vi "Force Recorder.vi"() -> ()   [LabVIEW 2017]
uses:
  <vilib>/Platform/TimedLoop/XDataNode/timing_clust.ctl
  <vilib>/Platform/TimedLoop/XDataNode/nitl_modes.ctl
  <vilib>/Platform/TimedLoop/XDataNode/wakeup.ctl
  <vilib>/Utility/sysdir.llb/System Directory Type.ctl
  <vilib>/DAQmx/read.llb/DAQmx Read (Analog 1D DBL NChan 1Samp).vi
  <vilib>/Instr/_visa.llb/VISA Configure Serial Port (Instr).vi
  <vilib>/Utility/file.llb/Write Delimited Spreadsheet (string).vi
  <vilib>/Utility/file.llb/Write Delimited Spreadsheet (DBL).vi
  <vilib>/DAQmx/create/channels.llb/DAQmx Create Channel (AI-Voltage-Basic).vi
  <vilib>/DAQmx/configure/timing.llb/DAQmx Timing (Sample Clock).vi
  <vilib>/DAQmx/miscellaneous.llb/DAQmx Fill In Error Info.vi
  <vilib>/platform/TimedLoop/XDataNode/XDataNode.xnode
  <vilib>/Platform/TimedLoop/XDataNode/XDNodeRunTimeDep.lvlib
panel:
  out "FW Up":i32
  out "RW Down":i32
  out "RW Up":i32
  out "FW Down":i32
  out "Loop":i32
  out "Save in Time":dbl[][](array[numeric])
  out "SaveReady":bool
  out "RW Force Up":T1
  out "FW Force Up":T1
  out "RW Force Down":T1
  out "FW Force Down":T1
  in  "Read":bool
  in  "Save Type":enum32{"Save in time", "Save by step force"}(radio) caption="Save By Step Force"
  out "Volt Meter 2":dbl(graph)=0.034576825000000005
  in  "SAVE":bool
  out "Save Path":path
  out "Volt Meter 1":dbl(graph)=0.0048819160000000035
  in  "Test Name":string(combo)="DL"
  in  "Lane Number":string(combo)="Lane 1"
  out "Force Meter":dbl(graph)=0.06621116599999999
  out "error out":errorcluster
  in  "stop":bool
  out "Serial OK":bool
  out "Step Force":u8[](array[numeric])
  in  "Serial Port":refnum<visa-resource-name>="COM3"
  in  "Baud Rate":string(combo)="19200"
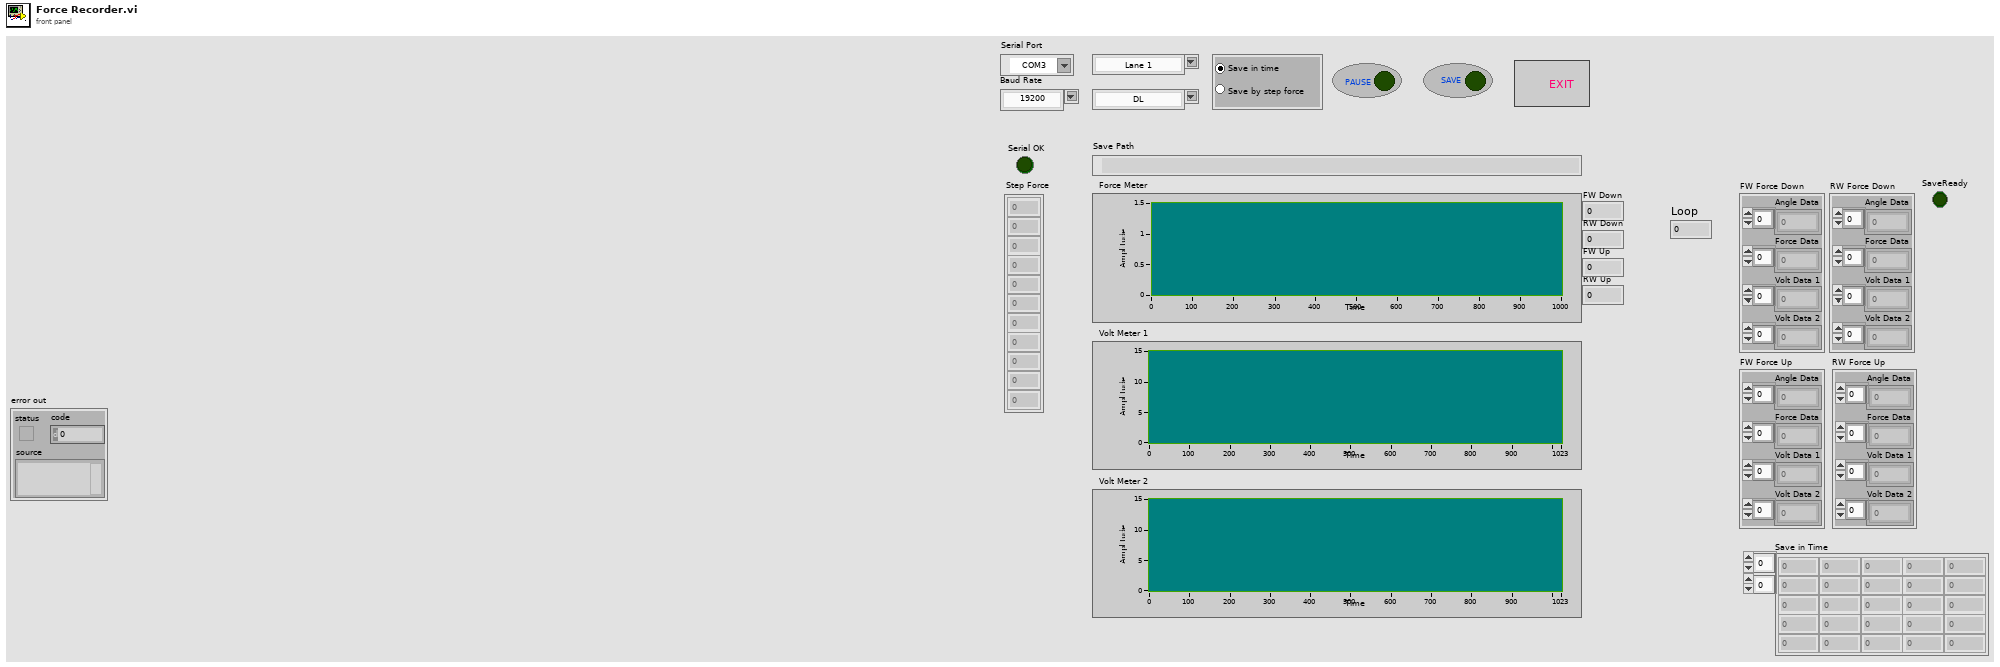
[diagram p1: front panel]
types:
  T1 = cluster{"Angle Data":dbl[], "Force Data":dbl[], "Volt Data 1":dbl[], "Volt Data 2":dbl[]}
  T2 = cluster{"Angle":dbl[], "Force":dbl[], "Volt 1":dbl[], "Volt 2":dbl[]}
  T3 = typedef "XDNodeRunTimeDep.lvlib/timing_clust.ctl" = cluster{"Expected End [f-1]":u64, "Actual End [f-1]":u64, "Finished Late? [f-1]":bool, "Expected End [i-1]":u64, "Actual End [i-1]":u64, "Finished Late? [i-1]":bool, "Expected Start [i]":u64, "Actual Start [i]":u64, "Expected Start [f]":u64, "Actual Start [f]":u64, "Source Name":string, "Structure Name":string, "Period":i64, "Deadline":i64, "Offset":i64, "Start":i64, "Priority":i32, "Timeout":i32, "Mode":T4, "Wakeup Reason":T5, "Error":errorcluster, "Source Type":string, "Secondary Source Type":string, "Global End Time":u64, "Global Start Time":u64, "Frame Duration":u64, "Iteration Duration":u64, "Assigned CPU":i32, "I/O Scan Engine Mode":u32}
  T4 = typedef "XDNodeRunTimeDep.lvlib/nitl_modes.ctl" = enum32{"No Change", "Process missed periods, maintain original phase", "Discard missed periods, maintain original phase", "Process missed periods, ignore original phase", "Discard missed periods, ignore original phase"}
  T5 = typedef "XDNodeRunTimeDep.lvlib/wakeup.ctl" = enum32{"Normal", "Aborted", "Asynchronous wakeup", "Timing source error", "Timed loop error", "Timeout"}
  T6 = enum8{"Enabled", "Disabled", "Disabled and Grayed Out"}
  T7 = typedef "System Directory Type.ctl" = i32
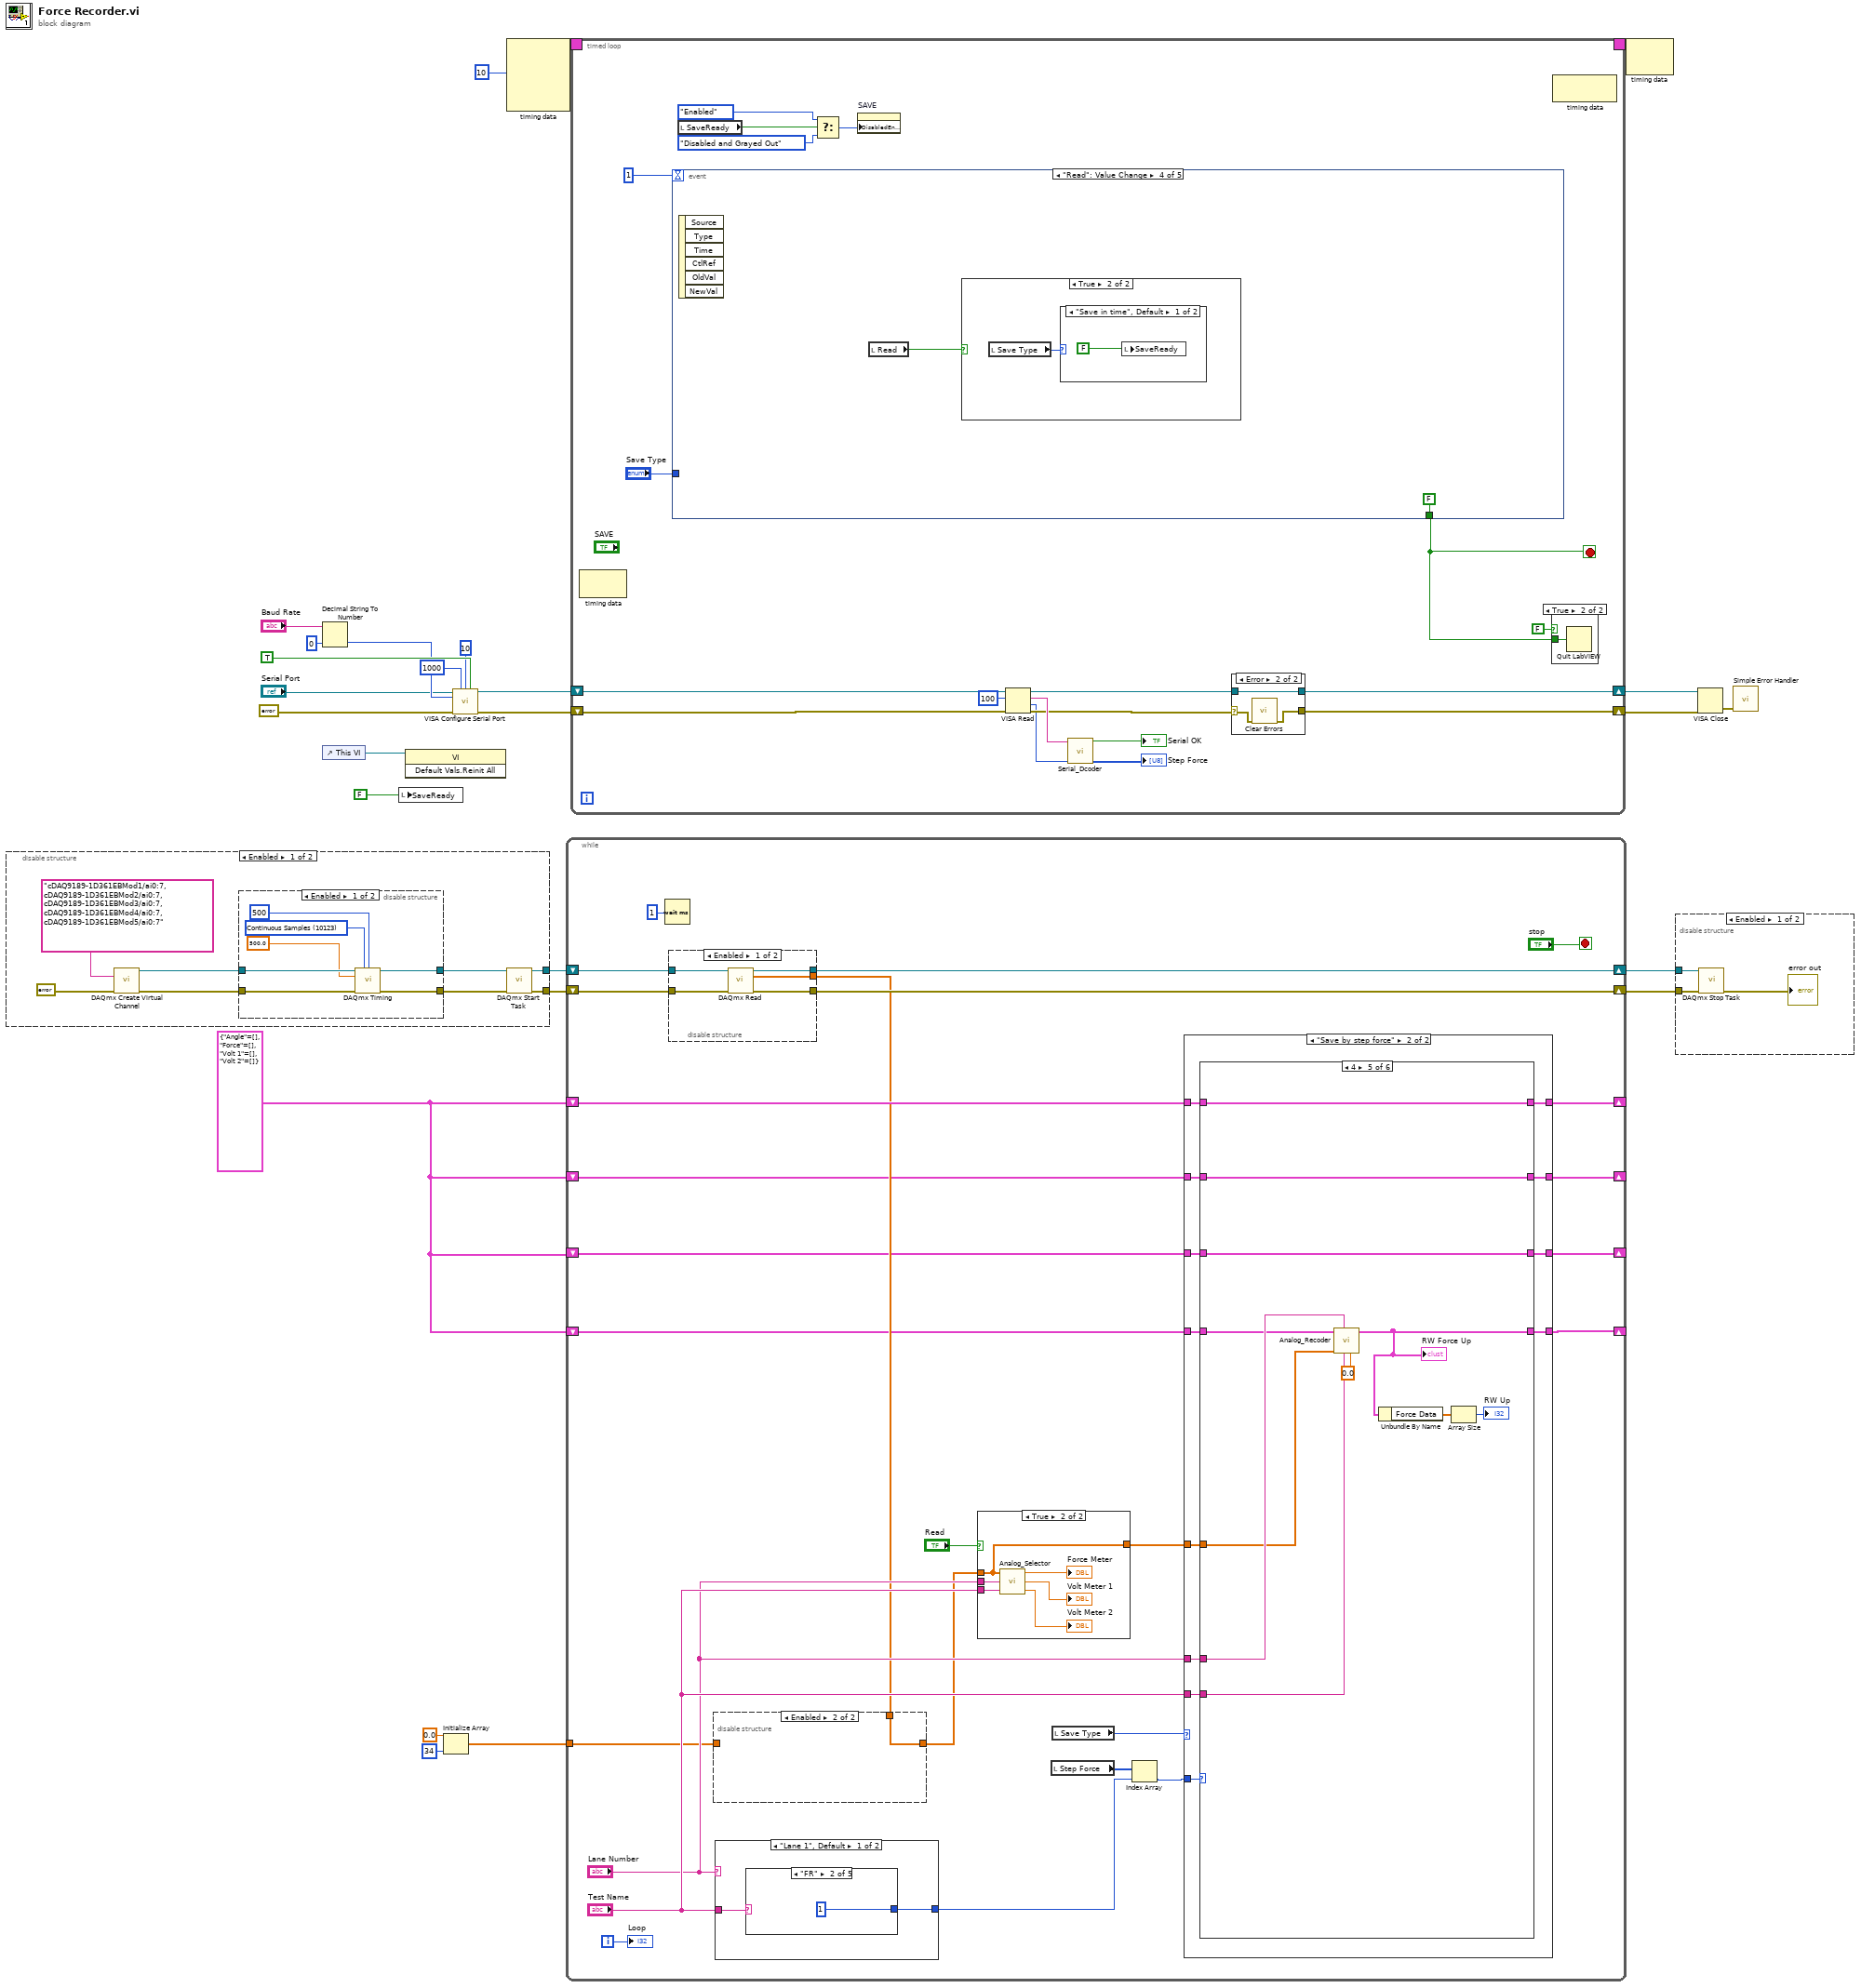
[diagram p0: block diagram]
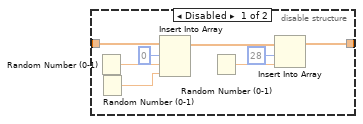
[diagram p2: hidden frame]
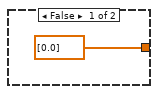
[diagram p3: hidden frame]
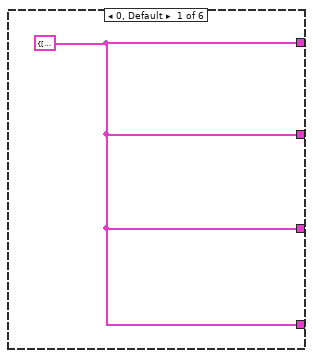
[diagram p5: hidden frame]
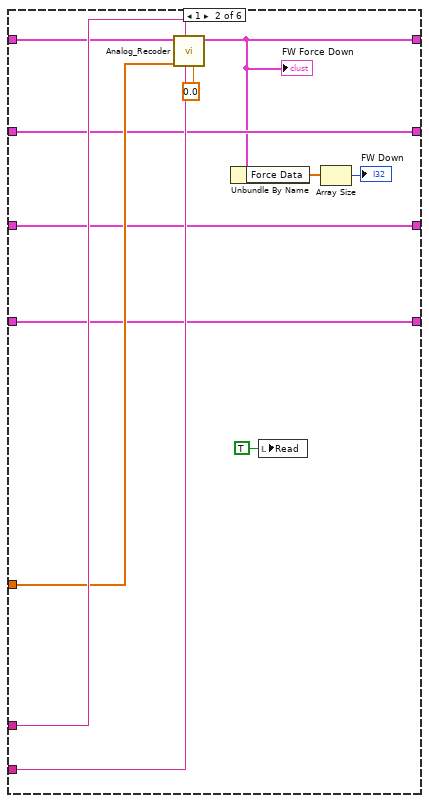
[diagram p6: hidden frame]
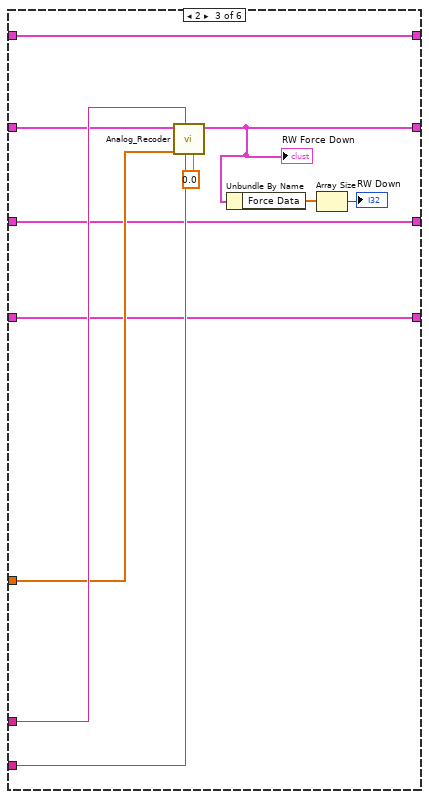
[diagram p7: hidden frame]
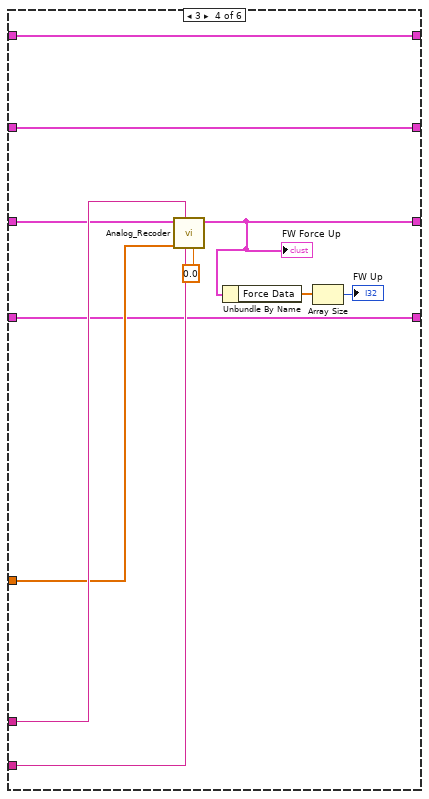
[diagram p8: hidden frame]
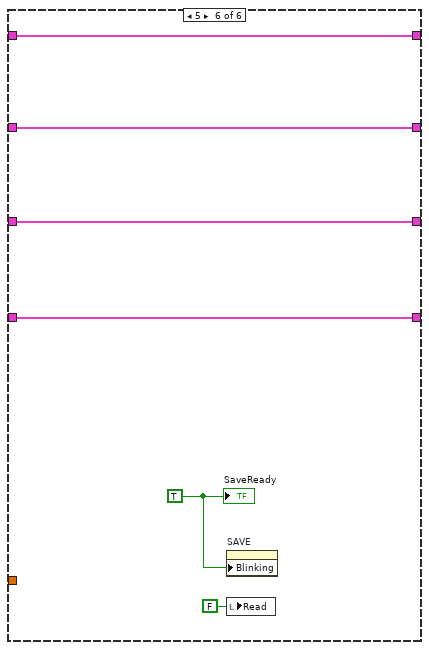
[diagram p9: hidden frame]
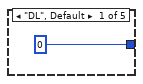
[diagram p11: hidden frame]
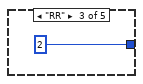
[diagram p12: hidden frame]
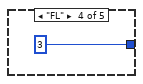
[diagram p13: hidden frame]
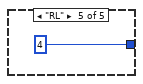
[diagram p14: hidden frame]
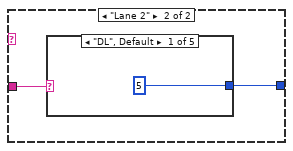
[diagram p15: hidden frame]
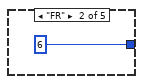
[diagram p16: hidden frame]
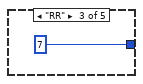
[diagram p17: hidden frame]
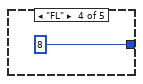
[diagram p18: hidden frame]
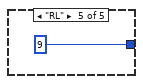
[diagram p19: hidden frame]
diagram:
  w2 = T2 {"Angle"=[], "Force"=[], "Volt 1"=[], "Volt 2"=[]}
  n1 = disable-structure shown="Enabled" {
    disable-tunnel: [w34 _] -> w9
    disable-tunnel: [w33 _] -> w8
    frame Enabled {
      n2 = call-poly <vilib>:"DAQmx Create Virtual Channel.vi"("physical channels"=tag "cDAQ9189-1D361EBMod1/ai0:7, cDAQ9189-1D361EBMod2/ai0:7, cDAQ9189-1D361EBMod3/ai0:7, cDAQ9189-1D361EBMod4/ai0:7, cDAQ9189-1D361EBMod5/ai0:7", "error in"=errorcluster {"status"=FALSE, "code"=0, "source"=""} ("error constant")) -> ("task out"=w30:refnum<k21>, "error out"=w29:errorcluster)  [unwired: 12 in]
      n3 = disable-structure shown="Enabled" {
        disable-tunnel: w30 -> [w41 w43]
        disable-tunnel: w29 -> [w40 w42]
        disable-tunnel: [w39 w43] -> w28
        disable-tunnel: [w38 w42] -> w27
        frame Enabled {
          w36 = 10123 items=["Finite Samples"=10178, "Continuous Samples"=10123, "Hardware Timed Single Point"=12522] ("sample mode")
          n4 = call-poly <vilib>:"DAQmx Timing.vi"("task/channels in"=w41, "sample mode"=w36, "samples per channel"=500, "rate"=500.0, "error in"=w40) -> ("task out"=w39:refnum<k21>, "error out"=w38:errorcluster)  [unwired: 9 in]
        }
        frame Disabled {
        }
      }
      n5 = call <vilib>:"DAQmx Start Task.vi"("task/channels in"=w28, "error in"=w27) -> ("task out"=w34:refnum<k21>, "error out"=w33:errorcluster)  [unwired: 12 in]
    }
    frame Disabled {
    }
  }
  n6 = Decimal String To Number(string="Baud Rate", default (0L)=u32 0 ("default (0 I32)")) -> (number=w18:u32)  [unwired: 1 in, 1 out]
  n7 = control-ref of="This VI"() -> (w10:refnum<vi>)
  n8 = local write "SaveReady"(FALSE ("SaveReady")) -> ()
  n9 = invoke class="VI" method="Default Vals.Reinit All"(reference=w10) -> ()  [unwired: 2 in, 3 out]
  n10 = Initialize Array(0.0 ("element"), 34 ("dimension size")) -> (w3:dbl[])
  n11 = call-poly "VISA Configure Serial Port"("VISA resource name"="Serial Port", "timeout (10sec)"=u32 1000, "termination char\n(0xA = '\\n' = LF)"=u8 10 ("termination char\n(0xA = '\\n' = LF)"), "Enable Termination\nChar (T)"=TRUE ("End Read on Termination Character?"), "baud rate (9600)"=w18, "error in (no error)"=errorcluster {"status"=FALSE, "code"=0, "source"=""}) -> ("VISA resource name out"=w16:refnum<visa-resource-name>, "error out"=w15:errorcluster)  [unwired: 4 in, 4 out]
  n12 = node-c288(i64 10 ("Period")) -> (w26:T3)  [unwired: 3 in]
  n13 = while {
    shift-right: [w63] -> w7
    shift-left: w9 -> [w65]
    shift-right: [w62] -> w6
    shift-left: w8 -> [w64]
    shift-right: [w68] -> _
    shift-left: w2 -> [w69]
    tunnel: w3 -> [w58]
    shift-right: [w53] -> _
    shift-left: w2 -> [w52]
    shift-right: [w50] -> _
    shift-left: w2 -> [w51]
    shift-right: [w49] -> _
    shift-left: w2 -> [w48]
    i -> [w47]
    stop <- "stop" stop-if-true
    n14 = Wait (ms)(milliseconds to wait=u32 1) -> ()  [unwired: 1 out]
    n15 = disable-structure shown="Enabled" {
      disable-tunnel: w65 -> [w158 _]
      disable-tunnel: w64 -> [w157 _]
      disable-tunnel: [w156 _] -> w63
      disable-tunnel: [w155 _] -> w62
      disable-tunnel: [w154 _] -> w55
      frame Enabled {
        n16 = call-poly <vilib>:"DAQmx Read.vi"("task/channels in"=w158, "error in"=w157) -> ("task out"=w156:refnum<k21>, "data"=w154:dbl[], "error out"=w155:errorcluster)  [unwired: 11 in]
      }
      frame Disabled {
      }
    }
    n17 = disable-structure shown="Enabled" {
      disable-tunnel: w58 -> [w73 _]
      disable-tunnel: [w70 w78] -> w56
      disable-tunnel: w55 -> [_ w78]
      frame Disabled {
        n18 = Random Number (0-1)() -> (number: 0 to 1=w75:dbl)
        n19 = Random Number (0-1)() -> (number: 0 to 1=w71:dbl)
        n20 = Insert Into Array(array=w73, index=0, new element #1=w75, new element #2=w71) -> (w72:dbl[])
        n21 = Random Number (0-1)() -> (number: 0 to 1=w76:dbl)
        n22 = Insert Into Array(array=w72, index=28, new element=w76) -> (w70:dbl[])
      }
      frame Enabled {
      }
    }
    n23 = case shown="\"Lane 1\", Default" "Lane Number" {
      tunnel: "Test Name" -> [w160 w167]
      tunnel: [w159 w166] -> w67
      frame "Lane 1", Default {
        n24 = case shown="\"FR\"" w160 {
          tunnel: [0 ("index") 1 ("index") 2 ("index") 3 ("index") 4 ("index")] -> w159
          frame "DL", Default {
          }
          frame "FR" {
          }
          frame "RR" {
          }
          frame "FL" {
          }
          frame "RL" {
          }
        }
      }
      frame "Lane 2" {
        n25 = case shown="\"DL\", Default" w167 {
          tunnel: [5 ("index") 6 ("index") 7 ("index") 8 ("index") 9 ("index")] -> w166
          frame "DL", Default {
          }
          frame "FR" {
          }
          frame "RR" {
          }
          frame "FL" {
          }
          frame "RL" {
          }
        }
      }
    }
    n26 = case shown="True" "Read" {
      tunnel: "Test Name" -> [_ w82]
      tunnel: "Lane Number" -> [_ w81]
      tunnel: w56 -> [_ w80]
      tunnel: [dbl[] [0.0] w80] -> w54
      frame False {
      }
      frame True {
        n27 = call "Analog_Selector.vi"("Test Name"=w82, "Lane Number"=w81, "Analog Data In"=w80) -> ("Volt 2"=→"Volt Meter 2":dbl, "Volt 1"=→"Volt Meter 1":dbl, "Force"=→"Force Meter":dbl)
      }
    }
    n28 = local read "Step Force"() -> (w66:u8[])
    n29 = local read "Save Type"() -> (w59:enum32{"Save in time", "Save by step force"})
    n30 = Index Array(array=w66, index=w67) -> (element=w44:u8)
    n31 = case shown="\"Save by step force\"" w59 {
      tunnel: w69 -> [w89 w101]
      tunnel: [w89 w100] -> w68
      tunnel: w54 -> [_ w99]
      tunnel: w44 -> [_ w98]
      tunnel: "Test Name" -> [_ w97]
      tunnel: "Lane Number" -> [_ w96]
      tunnel: [w88 w95] -> w53
      tunnel: w52 -> [w88 w94]
      tunnel: w51 -> [w87 w93]
      tunnel: [w87 w92] -> w50
      tunnel: [w86 w91] -> w49
      tunnel: w48 -> [w86 w90]
      frame "Save in time", Default {
      }
      frame "Save by step force" {
        n32 = case shown="4" w98 {
          tunnel: w101 -> [_ w111 w118 w131 w143 w153]
          tunnel: [w102 w105 w118 w131 w143 w153] -> w100
          tunnel: w99 -> [_ w112 w123 w134 w145 _]
          tunnel: w97 -> [_ w113 w124 w135 w146 _]
          tunnel: w96 -> [_ w114 w125 w136 w147 _]
          tunnel: [w102 w109 w115 w129 w142 w152] -> w95
          tunnel: w94 -> [_ w109 w119 w129 w142 w152]
          tunnel: [w102 w108 w121 w126 w141 w151] -> w92
          tunnel: w93 -> [_ w108 w121 w130 w141 w151]
          tunnel: [w102 w107 w120 w132 w137 w150] -> w91
          tunnel: w90 -> [_ w107 w120 w132 w140 w150]
          frame 0, Default {
            w102 = T2 {"Angle"=[], "Force"=[], "Volt 1"=[], "Volt 2"=[]}
          }
          frame 1 {
            n33 = call "Analog_Recoder.vi"("External Angle In"=0.0, "Test Name"=w113, "Lane Number"=w114, "Analog Data In"=w112, "Analog Array In"=w111) -> ("Analog Array Out"=w105:T1)  [unwired: 6 in]
            "FW Force Down" <- w105
            n34 = Unbundle By Name(w105) -> ("Force Data"=w104:dbl[])
            n35 = local write "Read"(TRUE ("Read")) -> ()
            n36 = Array Size(array=w104) -> (size(s)=→"FW Down":i32)
          }
          frame 2 {
            n37 = call "Analog_Recoder.vi"("External Angle In"=0.0, "Test Name"=w124, "Lane Number"=w125, "Analog Data In"=w123, "Analog Array In"=w119) -> ("Analog Array Out"=w115:T1)  [unwired: 6 in]
            "RW Force Down" <- w115
            n38 = Unbundle By Name(w115) -> ("Force Data"=w117:dbl[])
            n39 = Array Size(array=w117) -> (size(s)=→"RW Down":i32)
          }
          frame 3 {
            n40 = call "Analog_Recoder.vi"("External Angle In"=0.0, "Test Name"=w135, "Lane Number"=w136, "Analog Data In"=w134, "Analog Array In"=w130) -> ("Analog Array Out"=w126:T1)  [unwired: 6 in]
            "FW Force Up" <- w126
            n41 = Unbundle By Name(w126) -> ("Force Data"=w128:dbl[])
            n42 = Array Size(array=w128) -> (size(s)=→"FW Up":i32)
          }
          frame 4 {
            n43 = call "Analog_Recoder.vi"("External Angle In"=0.0, "Test Name"=w146, "Lane Number"=w147, "Analog Data In"=w145, "Analog Array In"=w140) -> ("Analog Array Out"=w137:T1)  [unwired: 6 in]
            "RW Force Up" <- w137
            n44 = Unbundle By Name(w137) -> ("Force Data"=w139:dbl[])
            n45 = Array Size(array=w139) -> (size(s)=→"RW Up":i32)
          }
          frame 5 {
            w149 = TRUE ("SaveReady")
            n46 = property on="SAVE" class="Bool (strict)"("Blinking"=w149) -> ()  [unwired: 2 in, 2 out]
            n47 = local write "Read"(FALSE ("Read")) -> ()
            "SaveReady" <- w149
          }
        }
      }
    }
    "Loop" <- w47
  }
  n48 = timed-loop {
    timing: w26 -> [_]
    timing-out: [_] -> w25
    shift-right: [w191] -> w14
    shift-left: w16 -> [w184]
    shift-right: [w190] -> w13
    shift-left: w15 -> [w185]
    stop <- w173 stop-if-true
    n49 = node-c288() -> ()  [unwired: 1 in, 1 out]
    n50 = event shown="[3] \"Read\": Value Change" {
      selector: _ -> [_ _ _ _ _]
      dyn-events: _ -> [_ _ _ _ _]
      timeout: 1 -> [_ _ _ _ _]
      tunnel: [FALSE TRUE FALSE FALSE FALSE] -> w173
      tunnel: "Save Type" -> [_ _ w217 _ _]
      event Timeout {
        n51 = event-data() -> ()  [unwired: 1 in, 3 out]
      }
      event "stop": Value Change {
        n52 = event-data() -> ()  [unwired: 1 in, 3 out]
      }
      event "SAVE": Value Change {
        w197 = "_" ("string")
        w216 = T7 1 items=["User Home"=0, "User Desktop"=1, "User Documents"=2, "User Application Data"=3, "User Preferences"=4, "User Temporary"=5, "Public Documents"=6, "Public Application Data"=7, "Public Preferences"=8, "Public Cache"=13, "System Core Libraries"=9, "System Installed Libraries"=10, "Application Files"=11, "Boot Volume Root"=12] ("system directory type")
        n53 = event-data() -> ()  [unwired: 1 in, 6 out]
        n54 = local read "Lane Number"() -> (w205:string)
        n55 = local read "Test Name"() -> (w204:string)
        n56 = local write "SaveReady"(FALSE ("SaveReady")) -> ()
        n57 = Get Date/Time String(date format (0)=enum16{"short", "long", "abbreviated"}."short", want seconds? (F)=TRUE) -> (date string=w210:string, time string=w199:string)  [unwired: 1 in]
        n58 = Search and Replace String(replace all?=TRUE ("replace all? (F)"), input string=w210, search string="/", replace string="-" ("replace string (\"\")")) -> (result string=w206:string)  [unwired: 4 in, 3 out]
        n59 = Search and Replace String(replace all?=TRUE ("replace all? (F)"), input string=w199, search string=":", replace string="") -> (result string=w198:string)  [unwired: 4 in, 3 out]
        n60 = call <vilib>:"Get System Directory.vi"("system directory type"=w216) -> ("system directory"=w215:path)  [unwired: 10 in]
        n61 = Path To String(path=w215) -> (string=w214:string)
        n62 = Concatenate Strings(w214, "\\" ("string"), "ForceLog_" ("string"), w206, w197, w198, w197, w205, w197, w204) -> (w194:string)
        n63 = property on="SAVE" class="Bool (strict)"("Blinking"=FALSE) -> ()  [unwired: 2 in, 2 out]
        n64 = case shown="\"Save by step force\"" w217 {
          tunnel: w194 -> [w219 w243]
          frame "Save in time", Default {
            n65 = stacked-sequence {
              tunnel: w219 -> [w220 w232]
              frame #0 {
                n66 = Concatenate Strings(w220, ".csv" ("string")) -> (w222:string)
                n67 = String To Path(string=w222) -> (path=w221:path)
                n68 = call-poly <vilib>:"Write Delimited Spreadsheet.vi"("file path (dialog if empty)"=w221, "2D data"=string[][] [["Angle", "Force", "Volt 1", "Volt 2"]], "append to file? (new file:F)"=TRUE, "transpose? (no:F)"=FALSE, "delimiter (\\t)"="," ("delimiter (\\t)")) -> ()  [unwired: 9 in, 2 out]
              }
              frame #1 {
                n69 = property on="Force Meter" class="WFChart (strict)"() -> ("History Data"=w236:dbl[])  [unwired: 2 in, 2 out]
                n70 = property on="Volt Meter 1" class="WFChart (strict)"() -> ("History Data"=w235:dbl[])  [unwired: 2 in, 2 out]
                n71 = property on="Volt Meter 2" class="WFChart (strict)"() -> ("History Data"=w234:dbl[])  [unwired: 2 in, 2 out]
                n72 = Concatenate Strings(w232, ".csv" ("string")) -> (w230:string)
                n73 = String To Path(string=w230) -> (path=w229:path)
                n74 = Build Array(dbl[] [0.0] ("element"), w236, w235, w234) -> (w241:dbl[][])
                "Save in Time" <- w241
                n75 = Transpose 2D Array(2D array=w241) -> (transposed array=w242:dbl[][])
                n76 = call-poly <vilib>:"Write Delimited Spreadsheet.vi"("file path (dialog if empty)"=w229, "format (%.3f)"="%.6f", "2D data"=w242, "append to file? (new file:F)"=TRUE, "transpose? (no:F)"=FALSE, "delimiter (\\t)"="," ("delimiter (\\t)")) -> ("new file path (Not A Path if cancelled)"=→"Save Path":path)  [unwired: 8 in, 1 out]
              }
            }
          }
          frame "Save by step force" {
            n77 = stacked-sequence {
              tunnel: w243 -> [w244 w252 w260 w268 w284 w298 w312 w326]
              frame #0 {
                n78 = Concatenate Strings(w244, "_FW_Down.csv" ("string")) -> (w247:string)
                n79 = String To Path(string=w247) -> (path=w245:path)
                n80 = call-poly <vilib>:"Write Delimited Spreadsheet.vi"("file path (dialog if empty)"=w245, "2D data"=string[][] [["Angle", "Force", "Volt 1", "Volt 2"]], "append to file? (new file:F)"=FALSE, "transpose? (no:F)"=FALSE, "delimiter (\\t)"="," ("delimiter (\\t)")) -> ()  [unwired: 9 in, 2 out]
              }
              frame #1 {
                n81 = Concatenate Strings(w252, "_RW_Down.csv" ("string")) -> (w255:string)
                n82 = String To Path(string=w255) -> (path=w253:path)
                n83 = call-poly <vilib>:"Write Delimited Spreadsheet.vi"("file path (dialog if empty)"=w253, "2D data"=string[][] [["Angle", "Force", "Volt 1", "Volt 2"]], "append to file? (new file:F)"=FALSE, "transpose? (no:F)"=FALSE, "delimiter (\\t)"="," ("delimiter (\\t)")) -> ()  [unwired: 9 in, 2 out]
              }
              frame #2 {
                n84 = Concatenate Strings(w260, "_FW_Up.csv" ("string")) -> (w263:string)
                n85 = String To Path(string=w263) -> (path=w261:path)
                n86 = call-poly <vilib>:"Write Delimited Spreadsheet.vi"("file path (dialog if empty)"=w261, "2D data"=string[][] [["Angle", "Force", "Volt 1", "Volt 2"]], "append to file? (new file:F)"=FALSE, "transpose? (no:F)"=FALSE, "delimiter (\\t)"="," ("delimiter (\\t)")) -> ()  [unwired: 9 in, 2 out]
              }
              frame #3 {
                n87 = Concatenate Strings(w268, "_RW_Up.csv" ("string")) -> (w271:string)
                n88 = String To Path(string=w271) -> (path=w269:path)
                n89 = call-poly <vilib>:"Write Delimited Spreadsheet.vi"("file path (dialog if empty)"=w269, "2D data"=string[][] [["Angle", "Force", "Volt 1", "Volt 2"]], "append to file? (new file:F)"=FALSE, "transpose? (no:F)"=FALSE, "delimiter (\\t)"="," ("delimiter (\\t)")) -> ()  [unwired: 9 in, 2 out]
              }
              frame #4 {
                n90 = local read "FW Force Down"() -> (w283:T1)
                n91 = Unbundle By Name(w283) -> ("Angle Data"=w282:dbl[], "Force Data"=w281:dbl[], "Volt Data 1"=w280:dbl[], "Volt Data 2"=w279:dbl[])
                n92 = Concatenate Strings(w284, "_FW_Down.csv" ("string")) -> (w286:string)
                n93 = String To Path(string=w286) -> (path=w285:path)
                n94 = Build Array(w282, w281, w280, w279) -> (w278:dbl[][])
                n95 = Transpose 2D Array(2D array=w278) -> (transposed array=w276:dbl[][])
                n96 = call-poly <vilib>:"Write Delimited Spreadsheet.vi"("file path (dialog if empty)"=w285, "2D data"=w276, "append to file? (new file:F)"=TRUE, "transpose? (no:F)"=FALSE, "delimiter (\\t)"="," ("delimiter (\\t)")) -> ()  [unwired: 9 in, 2 out]
              }
              frame #5 {
                n97 = local read "RW Force Down"() -> (w290:T1)
                n98 = Unbundle By Name(w290) -> ("Angle Data"=w297:dbl[], "Force Data"=w296:dbl[], "Volt Data 1"=w295:dbl[], "Volt Data 2"=w294:dbl[])
                n99 = Concatenate Strings(w298, "_RW_Down.csv" ("string")) -> (w300:string)
                n100 = String To Path(string=w300) -> (path=w299:path)
                n101 = Build Array(w297, w296, w295, w294) -> (w293:dbl[][])
                n102 = Transpose 2D Array(2D array=w293) -> (transposed array=w292:dbl[][])
                n103 = call-poly <vilib>:"Write Delimited Spreadsheet.vi"("file path (dialog if empty)"=w299, "2D data"=w292, "append to file? (new file:F)"=TRUE, "transpose? (no:F)"=FALSE, "delimiter (\\t)"="," ("delimiter (\\t)")) -> ()  [unwired: 9 in, 2 out]
              }
              frame #6 {
                n104 = local read "FW Force Up"() -> (w304:T1)
                n105 = Unbundle By Name(w304) -> ("Angle Data"=w311:dbl[], "Force Data"=w310:dbl[], "Volt Data 1"=w309:dbl[], "Volt Data 2"=w308:dbl[])
                n106 = Concatenate Strings(w312, "_FW_Up.csv" ("string")) -> (w314:string)
                n107 = String To Path(string=w314) -> (path=w313:path)
                n108 = Build Array(w311, w310, w309, w308) -> (w307:dbl[][])
                n109 = Transpose 2D Array(2D array=w307) -> (transposed array=w306:dbl[][])
                n110 = call-poly <vilib>:"Write Delimited Spreadsheet.vi"("file path (dialog if empty)"=w313, "2D data"=w306, "append to file? (new file:F)"=TRUE, "transpose? (no:F)"=FALSE, "delimiter (\\t)"="," ("delimiter (\\t)")) -> ()  [unwired: 9 in, 2 out]
              }
              frame #7 {
                n111 = local read "RW Force Up"() -> (w318:T1)
                n112 = Unbundle By Name(w318) -> ("Angle Data"=w325:dbl[], "Force Data"=w324:dbl[], "Volt Data 1"=w323:dbl[], "Volt Data 2"=w322:dbl[])
                n113 = Concatenate Strings(w326, "_RW_Up.csv" ("string")) -> (w328:string)
                n114 = String To Path(string=w328) -> (path=w327:path)
                n115 = Build Array(w325, w324, w323, w322) -> (w321:dbl[][])
                n116 = Transpose 2D Array(2D array=w321) -> (transposed array=w320:dbl[][])
                n117 = call-poly <vilib>:"Write Delimited Spreadsheet.vi"("file path (dialog if empty)"=w327, "2D data"=w320, "append to file? (new file:F)"=TRUE, "transpose? (no:F)"=FALSE, "delimiter (\\t)"="," ("delimiter (\\t)")) -> ()  [unwired: 9 in, 2 out]
              }
            }
          }
        }
      }
      event "Read": Value Change {
        n118 = event-data() -> ()  [unwired: 1 in, 6 out]
        n119 = local read "Read"() -> (w333:bool)
        n120 = case shown="True" w333 {
          frame False {
            n121 = local write "SaveReady"(TRUE ("SaveReady")) -> ()
          }
          frame True {
            n122 = local read "Save Type"() -> (w335:enum32{"Save in time", "Save by step force"})
            n123 = case shown="\"Save in time\", Default" w335 {
              frame "Save in time", Default {
                n124 = local write "SaveReady"(FALSE ("SaveReady")) -> ()
              }
              frame "Save by step force" {
              }
            }
          }
        }
      }
      event "Save Type": Value Change {
        n125 = event-data() -> ()  [unwired: 1 in, 6 out]
        n126 = local write "SaveReady"(FALSE ("SaveReady")) -> ()
      }
    }
    n127 = local read "SaveReady"() -> (w177:bool)
    n128 = Select(t=T6."Enabled" ("Disabled"), s=w177, f=T6."Disabled and Grayed Out" ("Disabled")) -> (s? t:f=w176:T6)
    n129 = property on="SAVE" class="Bool (strict)"("DisabledEnum"=w176) -> ()  [unwired: 2 in, 2 out]
    n130 = VISA Read(VISA resource name=w184, byte count=u32 100, error in (no error)=w185) -> (VISA resource name out=w183:refnum<visa-resource-name>, read buffer=w187:string, return count=w181:u32, error out=w182:errorcluster)
    n131 = call "Serial_Dcoder.vi"("RX Count"=w181, "string"=w187) -> ("StepForce"=→"Step Force":u8[], "OK"=→"Serial OK":bool)  [unwired: 8 in]
    n132 = case shown="Error" w182 {
      selector: w182 -> [w340 w343]
      tunnel: w183 -> [w341 w344]
      tunnel: [w341 w344] -> w191
      tunnel: [w340 w342] -> w190
      frame No Error {
      }
      frame Error {
        n133 = call <vilib>:"Clear Errors.vi"("error in (no error)"=w343) -> ("error out"=w342:errorcluster)  [unwired: 5 in, 1 out]
      }
    }
    n134 = case shown="True" FALSE {
      tunnel: w173 -> [_ w339]
      frame False {
      }
      frame True {
        n135 = Quit LabVIEW(quit? (T)=w339) -> ()
      }
    }
    n136 = node-c288() -> ()  [unwired: 1 in, 1 out]
  }
  n137 = node-c288(w25) -> ()  [unwired: 1 out]
  n138 = disable-structure shown="Enabled" {
    disable-tunnel: w7 -> [w348 _]
    disable-tunnel: w6 -> [w347 _]
    frame Enabled {
      n139 = call <vilib>:"DAQmx Stop Task.vi"("task/channels in"=w348, "error in"=w347) -> ("error out"=→"error out":errorcluster)  [unwired: 12 in, 1 out]
    }
    frame Disabled {
    }
  }
  n140 = VISA Close(VISA resource name=w14, error in (no error)=w13) -> (error out=w24:errorcluster)
  n141 = call <vilib>:"Simple Error Handler.vi"("error in (no error)"=w24) -> ()  [unwired: 1 in, 8 out]
